vi "Has Destroyed.vi"(7 "Sender":refnum<class "Sender.lvclass">, 9 "Error":errorcluster, 10 "Actor":refnum<class "Actor.lvclass">, 11 "Has Destroyed in":refnum<class "Has Destroyed.lvclass">) -> (0 "Error out":errorcluster, 3 "Has Destroyed out":refnum<class "Has Destroyed.lvclass">)   [LabVIEW 2020, in "jettl.lvlib" / "Has Destroyed Msg.lvlib" / "Has Destroyed.lvclass"]
uses:
  Has Destroyed.lvclass
  Actor/Actor/Actor.lvclass
  Sender/Sender/Sender.lvclass
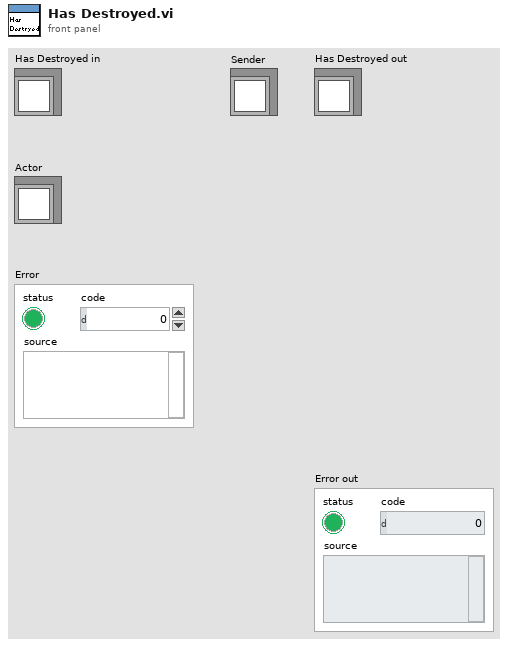
[diagram p1: front panel]
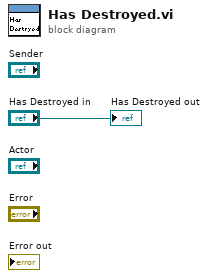
[diagram p0: block diagram]
diagram:
  "Has Destroyed out" <- "Has Destroyed in"
